vi "EjFGV.vi"() -> ()   [LabVIEW 2020]
doc: "Ejemplo de la variable global funcional"
uses:
  Abstract/Serial Device/Serial Device.lvclass
  Abstract/Serial Device/Serial Device.lvclass/Serial Device.ctl
panel:
  out "Visa com port":string
  out "data 2":string
  out "data":dbl
  in  "Numeric":dbl
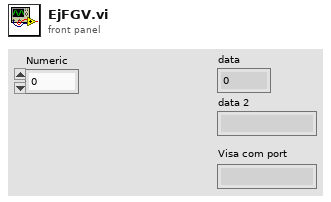
[diagram p1: front panel]
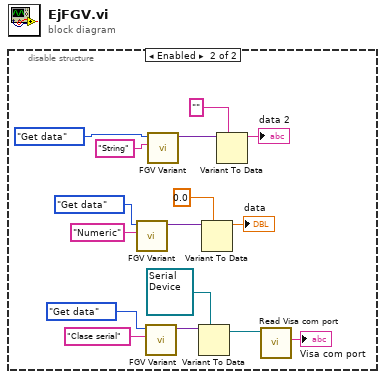
[diagram p0: block diagram]
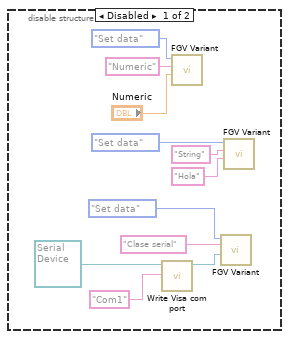
[diagram p2: hidden frame]
diagram:
  n1 = disable-structure shown="Enabled" {
    frame Disabled {
      n2 = call "Write Visa com port.vi"("Visa com port"="Com1", "Serial Device in"=refnum<class "Serial Device.lvclass"> refnum ("Serial Device.lvclass")) -> ("Serial Device out"=w3:refnum<class "Serial Device.lvclass">)  [unwired: 8 in, 1 out]
      n3 = call "FGV Variant.vi"("Data"="Numeric", "name"="Numeric", "Function"=enum16{"Reset data", "Get data", "Set data"}."Set data") -> ()  [unwired: 6 in, 3 out]
      n4 = call "FGV Variant.vi"("Data"=w3, "name"="Clase serial", "Function"=enum16{"Reset data", "Get data", "Set data"}."Set data") -> ()  [unwired: 6 in, 3 out]
      n5 = call "FGV Variant.vi"("Data"="Hola" ("name"), "name"="String", "Function"=enum16{"Reset data", "Get data", "Set data"}."Set data") -> ()  [unwired: 6 in, 3 out]
    }
    frame Enabled {
      n6 = call "FGV Variant.vi"("name"="Numeric", "Function"=enum16{"Reset data", "Get data", "Set data"}."Get data") -> ("value"=w24:variant)  [unwired: 7 in, 2 out]
      n7 = call "FGV Variant.vi"("name"="Clase serial", "Function"=enum16{"Reset data", "Get data", "Set data"}."Get data") -> ("value"=w15:variant)  [unwired: 7 in, 2 out]
      n8 = call "FGV Variant.vi"("name"="String", "Function"=enum16{"Reset data", "Get data", "Set data"}."Get data") -> ("value"=w26:variant)  [unwired: 7 in, 2 out]
      n9 = Variant To Data(type=refnum<class "Serial Device.lvclass"> refnum ("Serial Device out"), Variant=w15) -> (data=w13:refnum<class "Serial Device.lvclass">)  [unwired: 1 in, 1 out]
      n10 = Variant To Data(type=0.0 ("Numeric"), Variant=w24) -> (data=→"data":dbl)  [unwired: 1 in, 1 out]
      n11 = Variant To Data(type="" ("name"), Variant=w26) -> (data=→"data 2":string)  [unwired: 1 in, 1 out]
      n12 = call "Read Visa com port.vi"("Serial Device in"=w13) -> ("Visa com port"=→"Visa com port":string)  [unwired: 8 in, 2 out]
    }
  }
